vi "PXI-Get Delays.vi"(0 "Using Enhanced Alias Rejection":bool, 7 "AO Rate (Samples/s)":dbl, 9 "AI Rate (Samples/s)":dbl) -> (6 "AO delay (samples)":dbl, 10 "AI delay (samples)":dbl)   [LabVIEW 2020]
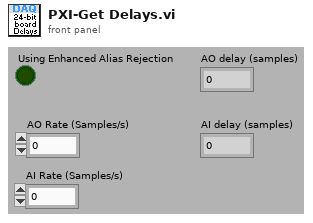
[diagram p1: front panel]
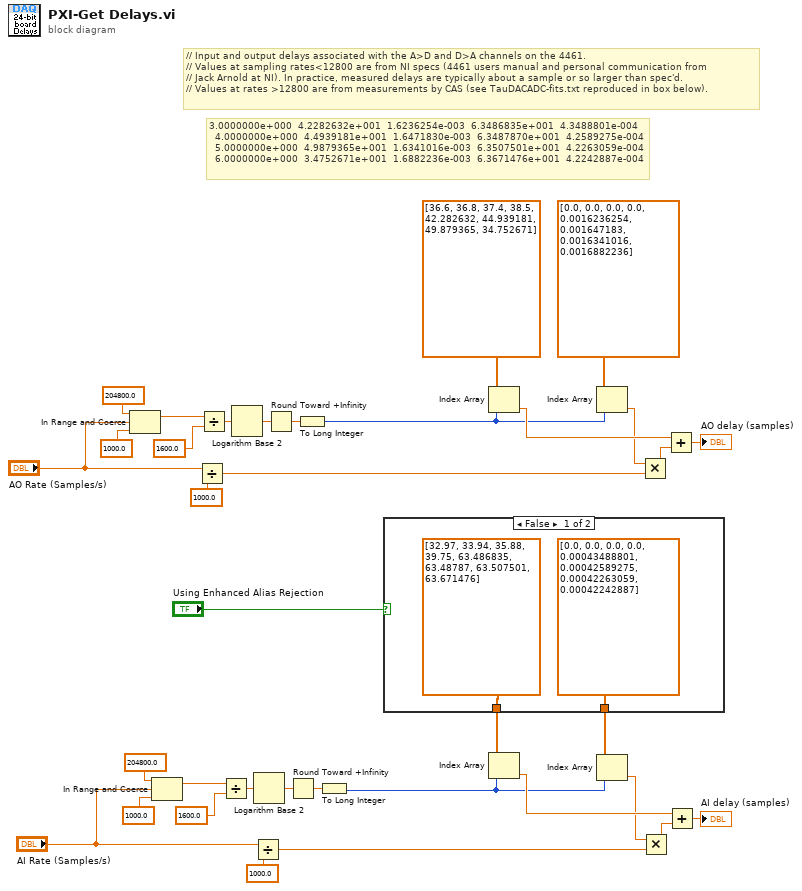
[diagram p0: block diagram]
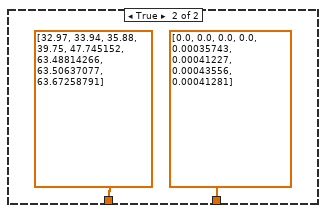
[diagram p2: hidden frame]
diagram:
  # "3.0000000e+000  4.2282632e+001  1.6236254e-003  6.3486835e+001  4.3488801e-004\n  4.0000000e+000  4.4939181e+001  1.6471830e-003  6.3487870e+001  4.2589275e-004\n  5.0000000e+000  4.9879365e+001  1.6341016e-003  6.3507501e+001  4.2263059e-004\n  6.0000000e+000  3.4752671e+001  1.6882236e-003  6.3671476e+001  4.2242887e-004"
  # "// Input and output delays associated with the A>D and D>A channels on the 4461.\n// Values at sampling rates<12800 are from NI specs (4461 users manual and personal communication from\n// Jack Arnold at NI). In practice, measured delays are typically about a sample or so larger than spec'd.\n// Values at rates >12800 are from measurements by CAS (see TauDACADC-fits.txt reproduced in box below)."
  n1 = In Range and Coerce(upper limit=204800.0, x="AO Rate (Samples/s)", lower limit=1000.0) -> (coerced(x)=w28:dbl)  [unwired: 1 out]
  n2 = In Range and Coerce(upper limit=204800.0, x="AI Rate (Samples/s)", lower limit=1000.0) -> (coerced(x)=w6:dbl)  [unwired: 1 out]
  n3 = Divide(x="AO Rate (Samples/s)", y=1000.0) -> (x/y=w4:dbl)
  n4 = Divide(x=w28, y=1600.0) -> (x/y=w31:dbl)
  n5 = Divide(x=w6, y=1600.0) -> (x/y=w9:dbl)
  n6 = Logarithm Base 2(1:w31) -> (0:w34:dbl)
  n7 = Divide(x="AI Rate (Samples/s)", y=1000.0) -> (x/y=w16:dbl)
  n8 = Logarithm Base 2(1:w9) -> (0:w12:dbl)
  n9 = Round Toward +Infinity(x=w34) -> (ceil(x): smallest int >= x=w33:dbl)
  n10 = Round Toward +Infinity(x=w12) -> (ceil(x): smallest int >= x=w11:dbl)
  n11 = To Long Integer(number=w33) -> (32bit integer=w20:i32)
  n12 = To Long Integer(number=w11) -> (32bit integer=w2:i32)
  n13 = case shown="False" "Using Enhanced Alias Rejection" {
    tunnel: [dbl[] [32.97, 33.94, 35.88, 39.75, 63.486835, 63.48787, 63.507501, 63.671476] ("array") dbl[] [32.97, 33.94, 35.88, 39.75, 47.745152, 63.48814266, 63.50637077, 63.67258791] ("array")] -> w27
    tunnel: [dbl[] [0.0, 0.0, 0.0, 0.0, 0.00043488801, 0.00042589275, 0.00042263059, 0.00042242887] ("array") dbl[] [0.0, 0.0, 0.0, 0.0, 0.00035743, 0.00041227, 0.00043556, 0.00041281] ("array")] -> w19
    frame False {
    }
    frame True {
    }
  }
  n14 = Index Array(array=dbl[] [36.6, 36.8, 37.4, 38.5, 42.282632, 44.939181, 49.879365, 34.752671], index=w20) -> (element=w23:dbl)
  n15 = Index Array(array=w27, index=w2) -> (element=w17:dbl)
  n16 = Index Array(array=dbl[] [0.0, 0.0, 0.0, 0.0, 0.0016236254, 0.001647183, 0.0016341016, 0.0016882236], index=w20) -> (element=w22:dbl)
  n17 = Index Array(array=w19, index=w2) -> (element=w15:dbl)
  n18 = Multiply(x=w22, y=w4) -> (x*y=w21:dbl)
  n19 = Multiply(x=w15, y=w16) -> (x*y=w18:dbl)
  n20 = Add(x=w23, y=w21) -> (x+y=→"AO delay (samples)":dbl)
  n21 = Add(x=w17, y=w18) -> (x+y=→"AI delay (samples)":dbl)
